vi "1.vi"() -> ()   [LabVIEW 2015]
panel:
  out "error out":errorcluster
  out "dup path":path
  in  "error in (no error)":errorcluster
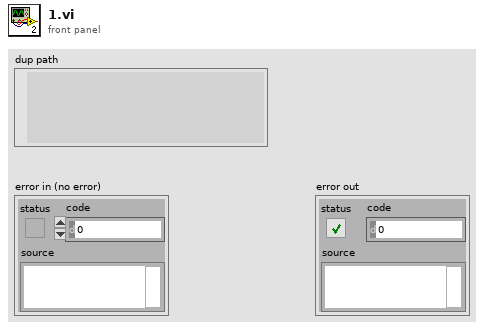
[diagram p1: front panel]
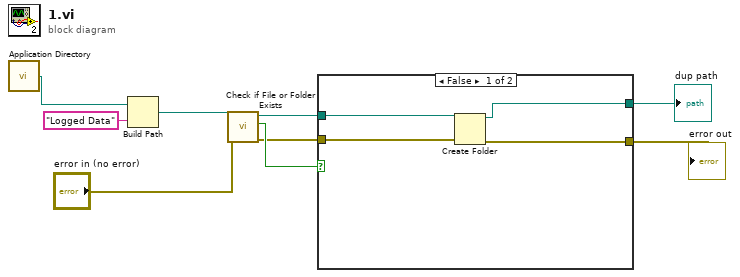
[diagram p0: block diagram]
diagram:
  n1 = call <vilib>:"Application Directory.vi"() -> ("Application Directory"=w9:path)
  n2 = Build Path(base path=w9, name or relative path="Logged Data") -> (appended path=w7:path)
  n3 = call <vilib>:"Check if File or Folder Exists.vi"("error in (no error)"="error in (no error)", "path"=w7) -> ("error out"=w3:errorcluster, "file or folder exists?"=w4:bool, "dup path"=w6:path)  [unwired: 7 in]
  n4 = case shown="False" w4 {
    tunnel: w6 -> [w13 w14]
    tunnel: w3 -> [w12 w15]
    tunnel: [w11 w15] -> w2
    tunnel: [w10 w14] -> w1
    frame False {
      n5 = Create Folder(path (use dialog)=w13, error in=w12) -> (created path=w10:path, error out=w11:errorcluster)  [unwired: 1 in, 1 out]
    }
    frame True {
    }
  }
  "dup path" <- w1
  "error out" <- w2
